vi "Write Grid.vi"(8 "error in (no error)":errorcluster, 10 "Grid":i16[][][](array[numeric]), 11 "CollisionGrid in":refnum<class "CollisionGrid.lvclass">) -> (0 "error out":errorcluster, 3 "CollisionGrid out":refnum<class "CollisionGrid.lvclass">)   [LabVIEW 2022 SP3, in "CollisionGrid.lvclass"]
uses:
  CollisionGrid.lvclass
  CollisionGrid.lvclass/CollisionGrid.ctl
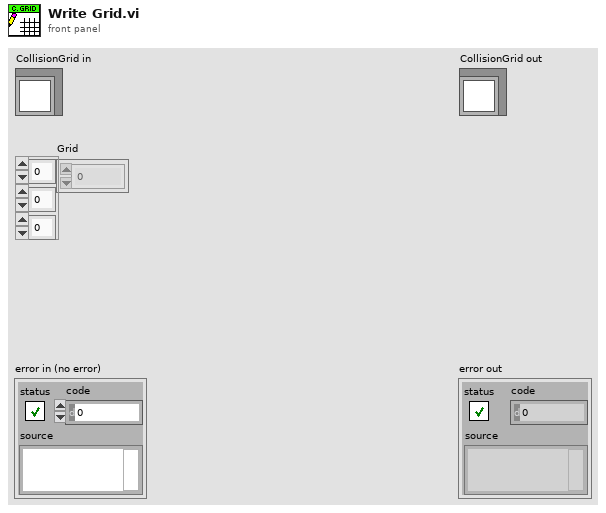
[diagram p1: front panel]
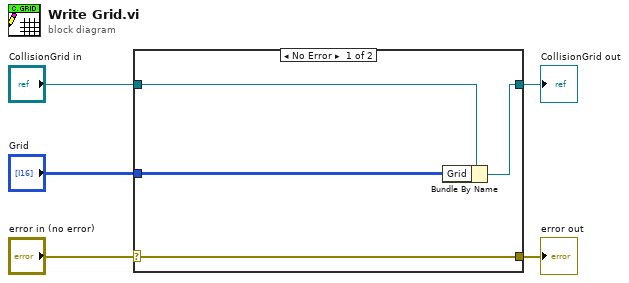
[diagram p0: block diagram]
diagram:
  n1 = case shown="No Error" "error in (no error)" {
    selector: "error in (no error)" -> [w9 w10]
    tunnel: [w9 w10] -> w4
    tunnel: [w7 w11] -> w2
    tunnel: "CollisionGrid in" -> [w8 w11]
    tunnel: "Grid" -> [w6 _]
    frame No Error {
      n2 = Bundle By Name(cluster=w8, "Grid"=w6) -> (w7:refnum<class "CollisionGrid.lvclass">)
    }
    frame Error {
    }
  }
  "error out" <- w4
  "CollisionGrid out" <- w2
